vi "GetImages.vi"(7 "Sim Image Index":i32=3, 8 "error in (no error)":errorcluster, 11 "MagSpec_Bella in":refnum<class "MagSpec_Bella.lvclass">) -> (0 "error out":errorcluster, 1 "output cluster":cluster{dbl[], dbl[]}[](graph), 3 "MagSpec_Bella out":refnum<class "MagSpec_Bella.lvclass">, 4 "Empty Image":bool[](array[boolean]))   [LabVIEW 2020, in "MagSpec_Bella.lvclass"]
uses:
  MagSpec_Bella.lvclass
  MagSpec_Bella.lvclass/MagSpec_Bella.ctl
  <vilib>/vision/NI_Vision_Development_Module.lvlib
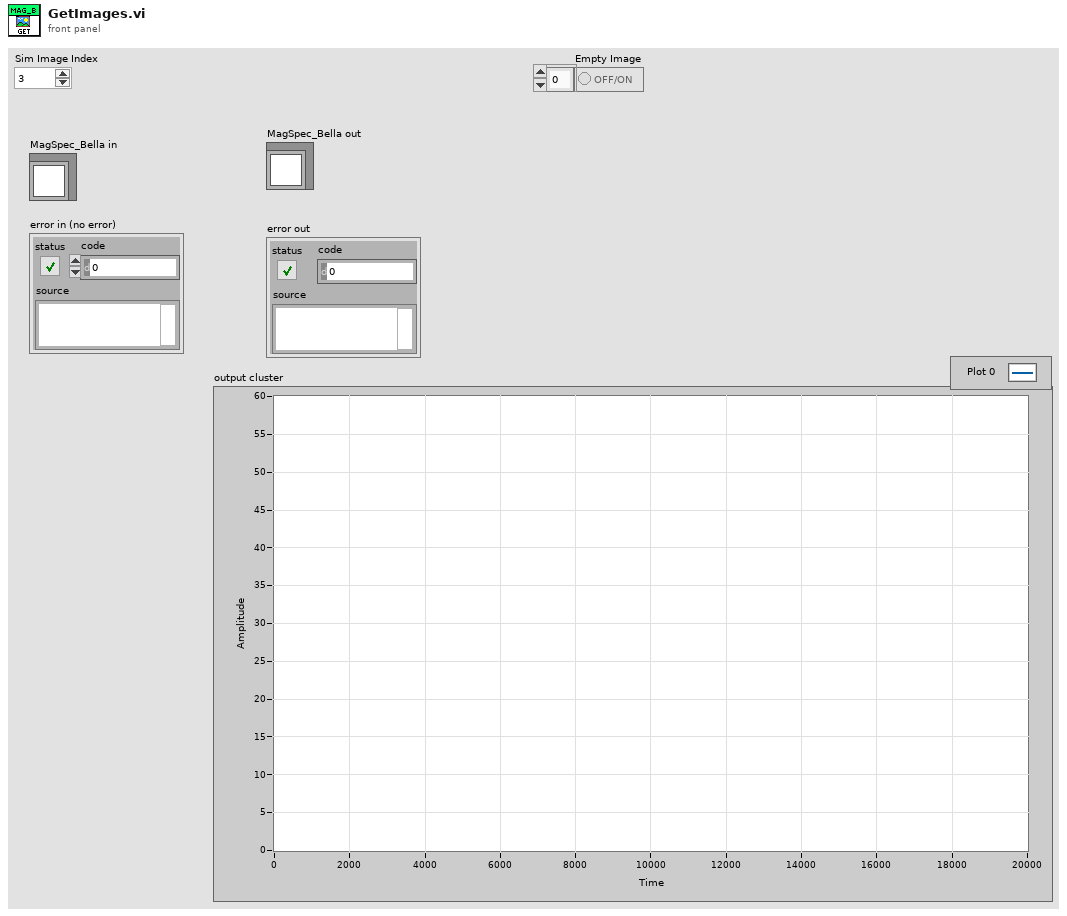
[diagram p1: front panel]
types:
  T1 = typedef "IMAQ Image.ctl" = refnum<image>
  T2 = typedef "Image Type" = u32
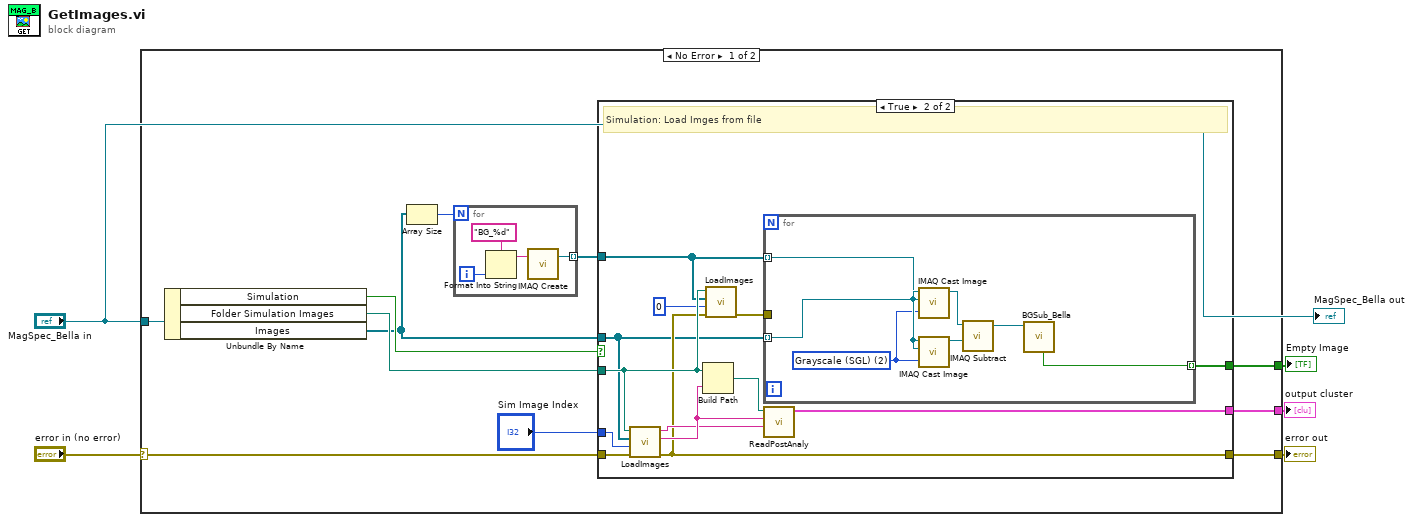
[diagram p0: block diagram]
diagram:
  n1 = case shown="No Error" "error in (no error)" {
    selector: "error in (no error)" -> [w14 w42]
    tunnel: "MagSpec_Bella in" -> [w16 _]
    tunnel: [w15 w42] -> w4
    tunnel: [w10 _] -> w3
    tunnel: [w6 _] -> w2
    frame No Error {
      n2 = Unbundle By Name(w16) -> ("Simulation"=w12:bool, "Folder Simulation Images"=w11:path, "Images"=w9:T1[])
      n3 = Array Size(array=w9) -> (size(s)=w8:i32)
      n4 = for {
        N: w8 -> [_]
        tunnel: [w17] -> w7 mode=indexing
        i -> [w20]
        n5 = Format Into String(format string="BG_%d", w20) -> (resulting string=w18:string)  [unwired: 2 in, 1 out]
        n6 = call "IMAQ Create"("Image Name"=w18) -> ("New Image"=w17:T1)  [unwired: 4 in, 1 out]
      }
      n7 = case shown="True" w12 {
        tunnel: w11 -> [_ w28]
        tunnel: w14 -> [w21 w34]
        tunnel: [w21 w26] -> w15
        tunnel: "Sim Image Index" -> [_ w33]
        tunnel: w9 -> [_ w25]
        tunnel: [_ w29] -> w10
        tunnel: w7 -> [_ w24]
        tunnel: [_ w22] -> w6
        frame False {
        }
        frame True {
          # "Simulation: Load Imges from file"
          n8 = call "LoadImages.vi"("error in (no error)"=w34, "Sim Image Index"=w33, "Images"=w25, "Folder Simulation Images"=w28) -> ("error out"=w26:errorcluster, "scan number"=w31:string, "shot number"=w30:string)  [unwired: 5 in]
          n9 = Build Path(base path=w28, name or relative path=w31) -> (appended path=w32:path)
          n10 = call "LoadImages.vi"("error in (no error)"=w26, "Sim Image Index"=0, "Images"=w24, "Folder Simulation Images"=w28) -> ("error out"=w23:errorcluster)  [unwired: 5 in, 2 out]
          n11 = for {
            tunnel: w25 -> [w40] mode=indexing
            tunnel: w24 -> [w37] mode=indexing
            tunnel: w23 -> [_]
            tunnel: [w36] -> w22 mode=indexing
            w35 = T2 2 items=["Grayscale (U8)", "Grayscale (I16)", "Grayscale (SGL)", "Complex (CSG)", "RGB (U32)", "HSL (U32)", "RGB (U64)", "Grayscale (U16)"] ("Image Type")
            n12 = call "IMAQ Cast Image"("Image Type"=w35, "Image Dst"=w40, "Image Src"=w40) -> ("Image Dst Out"=w39:T1)  [unwired: 7 in, 1 out]
            n13 = call "IMAQ Cast Image"("Image Type"=w35, "Image Dst"=w37, "Image Src"=w37) -> ("Image Dst Out"=w38:T1)  [unwired: 7 in, 1 out]
            n14 = call "IMAQ Subtract"("Image Src A"=w39, "Image Src B"=w38) -> ("Image Dst Out"=w41:T1)  [unwired: 5 in, 1 out]
            n15 = call "BGSub_Bella.vi"("raw Image In"=w41) -> ("empty image"=w36:bool)  [unwired: 7 in, 3 out]
          }
          n16 = call "ReadPostAnaly.vi"("shot number"=w30, "Scan"=w31, "folder path"=w32) -> ("output cluster"=w29:cluster{dbl[], dbl[]}[])  [unwired: 8 in]
        }
      }
    }
    frame Error {
    }
  }
  "error out" <- w4
  "output cluster" <- w3
  "Empty Image" <- w2
  "MagSpec_Bella out" <- "MagSpec_Bella in"
